vi "checkData.vi"(8 "error in (no error)":errorcluster, 11 "reference in":refnum<class "Notification Controller.lvclass">) -> (0 "error out":errorcluster, 3 "reference out":refnum<class "Notification Controller.lvclass">)   [LabVIEW 2014, in "Notification Controller.lvclass"]
uses:
  Notification Controller.lvclass
  APP/excelFile_class/fileType.ctl
  File Controller_llb/File Controller.lvclass
  APP/excelFile_class/excelFile.lvclass
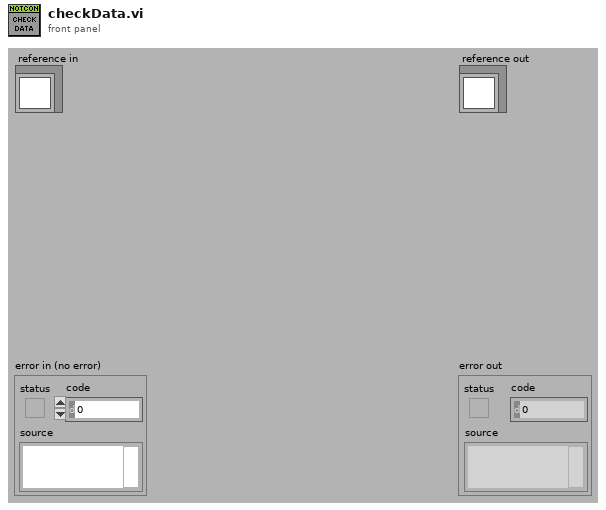
[diagram p1: front panel]
types:
  T1 = typedef "excelFile.lvclass/fileType.ctl" = enum16{"devices", "items", "partsTracking"}
  T2 = cluster{"second":i32, "minute":i32, "hour":i32, "day of month":i32, "month":i32, "year":i32, "day of week":i32, "day of year":i32, "is DST":i32}
  T3 = typedef "Notification Controller.lvclass/ObjectAttributesRef.ctl" = refnum<data-value>
  T4 = typedef "Notification Controller.lvclass/ObjectAttributes.ctl" = cluster{"MyAttribute":dbl, "items_data":string[][][], "items_notification_refs":refnum<class "itemsNotification.lvclass">[], "notifications_data_items":string[][], "items_nots?":bool, "devices_controller_ref":refnum<class "Devices Controller.lvclass">, "onlineUpdate":timestamp, "notController?":bool, "tracking_notification_ref":refnum<class "trackingNotification.lvclass">, "notifications_data_tracking":string[][], "tracking_parts_data":string[][], "tracking_nots?":bool, "index_tracking_not":i32[], "file_controller_ref":refnum<class "File Controller.lvclass">}
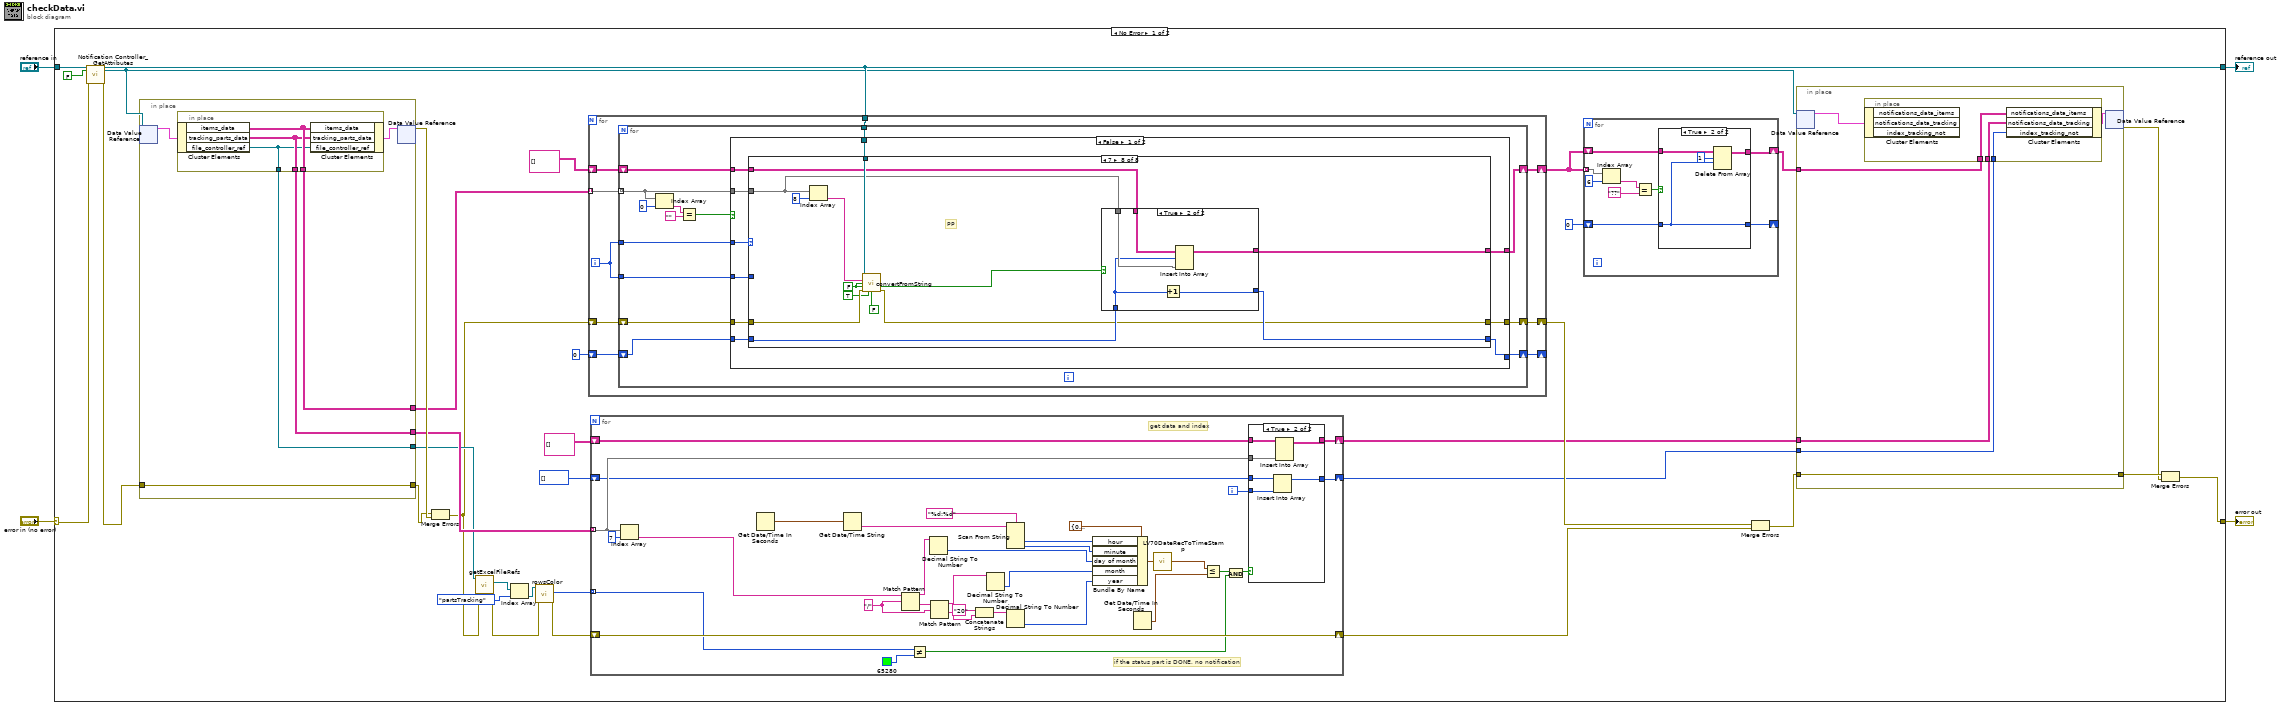
[diagram p0: block diagram]
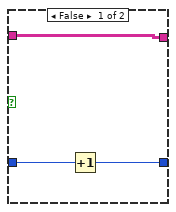
[diagram p3: hidden frame]
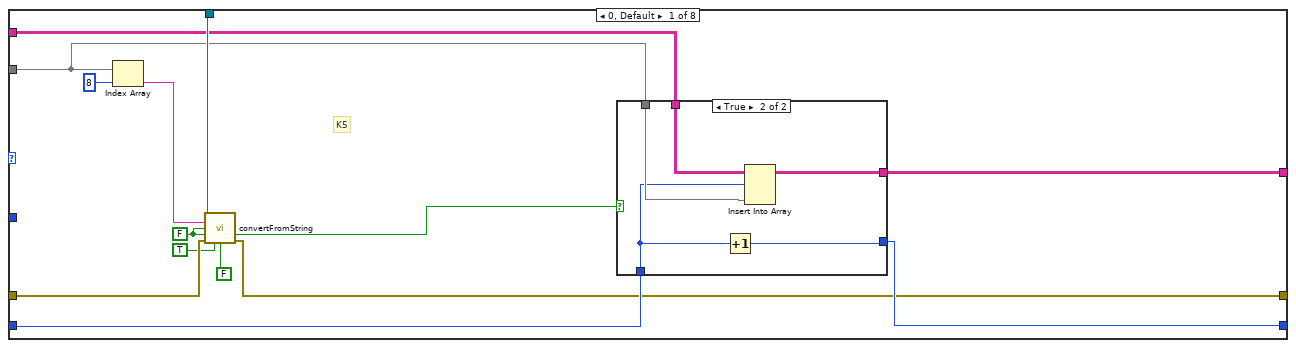
[diagram p4: hidden frame]
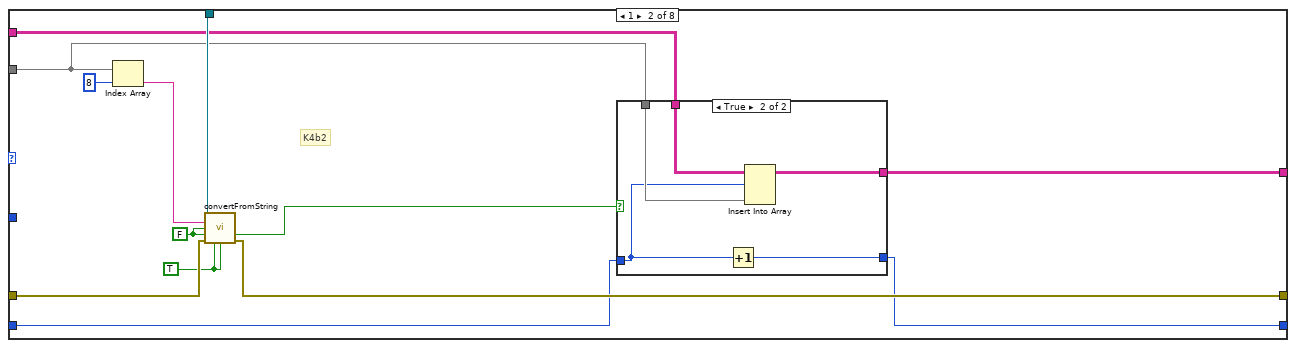
[diagram p6: hidden frame]
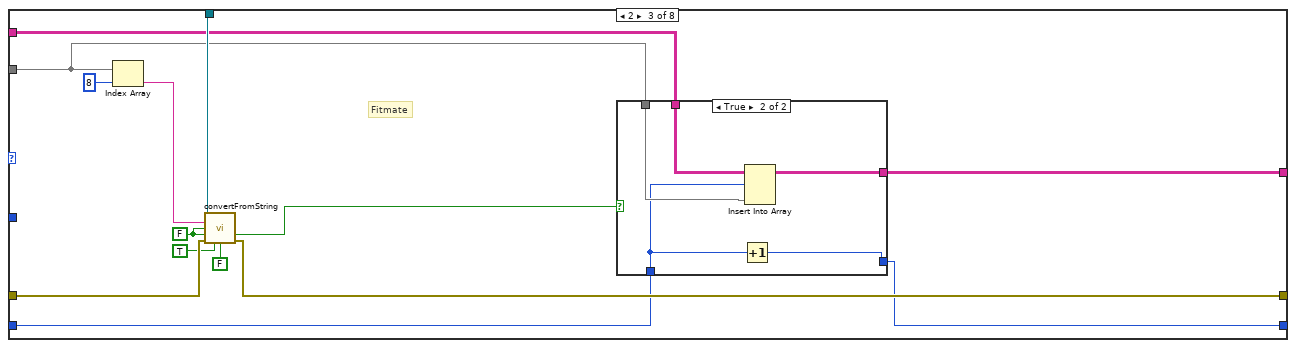
[diagram p8: hidden frame]
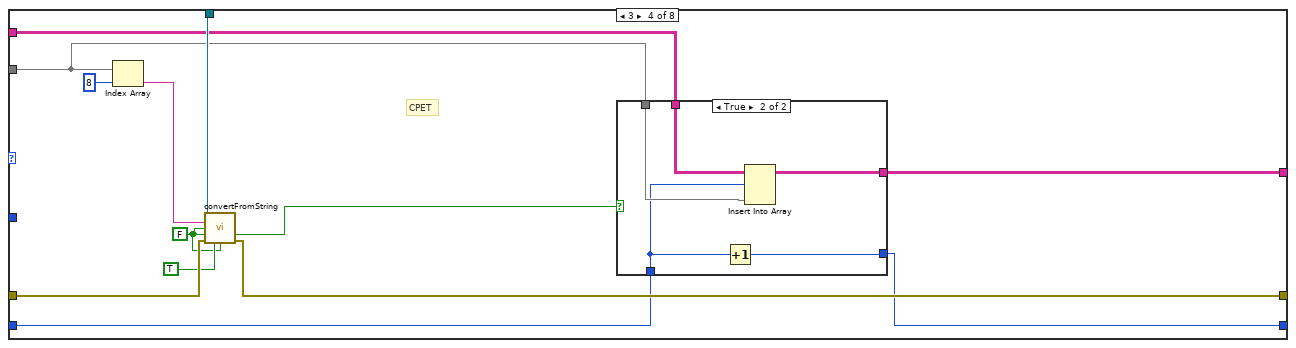
[diagram p10: hidden frame]
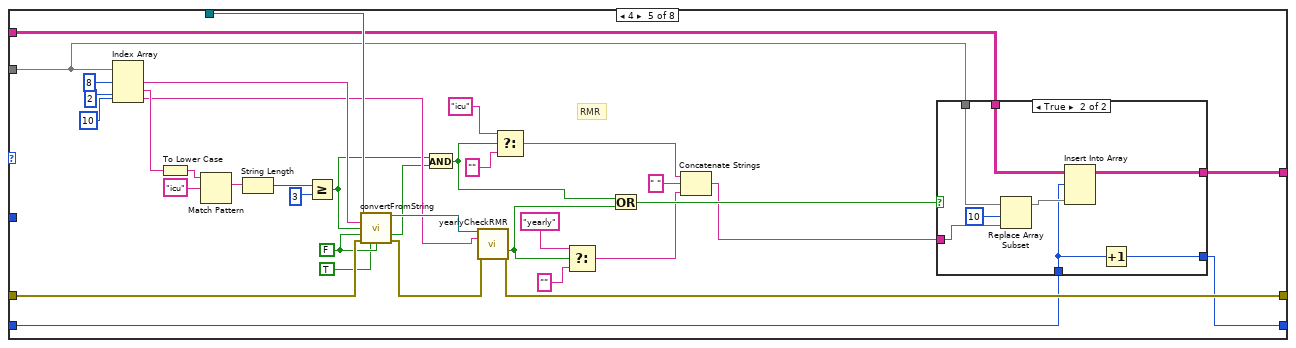
[diagram p12: hidden frame]
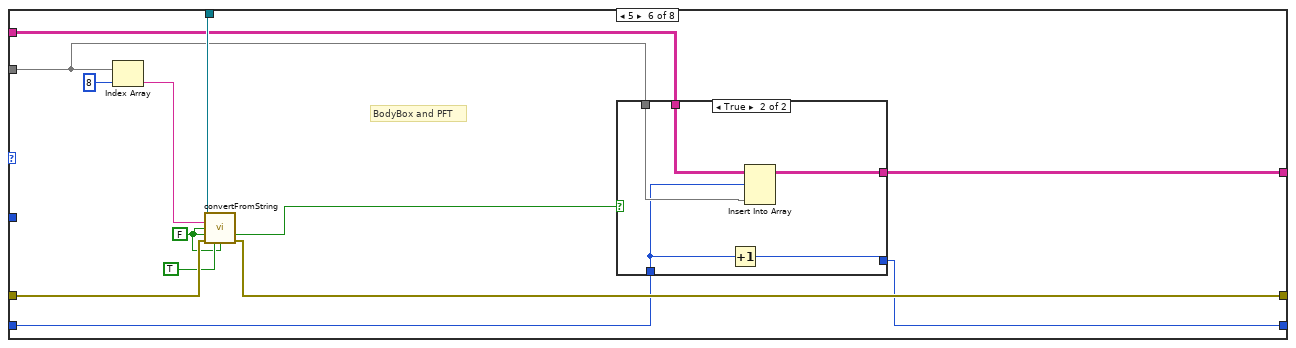
[diagram p14: hidden frame]
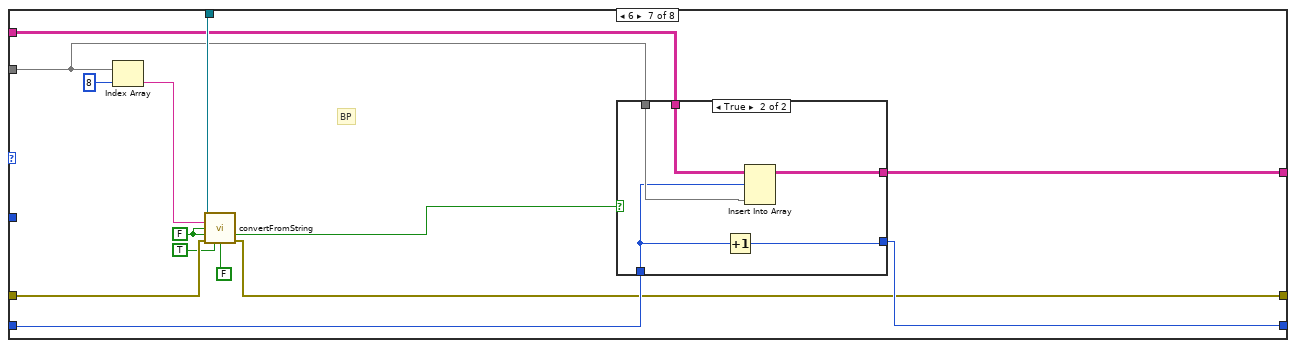
[diagram p16: hidden frame]
diagram:
  n1 = case shown="No Error" "error in (no error)" {
    selector: "error in (no error)" -> [w33 w340]
    tunnel: [w25 w340] -> w3
    tunnel: [w29 w339] -> w1
    tunnel: "reference in" -> [w35 w339]
    frame No Error {
      n2 = call "Notification Controller_GetAttributes.vi"("reference in"=w35, "return data? (T)"=FALSE, "error in (no error)"=w33) -> ("reference out"=w29:refnum<class "Notification Controller.lvclass">, "attributes ref"=w28:T3, "error out"=w32:errorcluster)  [unwired: 13 in, 1 out]
      n3 = in-place {
        in-place-border: w32 -> [w333]
        in-place-border: [w333] -> w36
        in-place-border: [w332] -> w30
        in-place-border: [w331] -> w20
        in-place-border: [w330] -> w12
        n4 = in-place-dvr #1(w28) -> (w334:T4)  [unwired: 1 out]
        n5 = in-place {
          in-place-border: [w338] -> w332
          in-place-border: [w337] -> w331
          in-place-border: [w336] -> w330
          n6 = in-place-cluster #2(w334) -> ("items_data"=w338:string[][][], "tracking_parts_data"=w337:string[][], "file_controller_ref"=w336:refnum<class "File Controller.lvclass">)
          n7 = in-place-cluster #2("items_data"=w338, "tracking_parts_data"=w337, "file_controller_ref"=w336) -> (w335:T4)
        }
        n8 = in-place-dvr #1(w335) -> (w37:errorcluster)  [unwired: 1 out]
      }
      n9 = Merge Errors(w36, w37) -> (w9:errorcluster)
      n10 = call "getExcelFileRefs.vi"("error in (no error)"=w9, "reference in"=w12) -> ("error out"=w5:errorcluster, "excelFile_refs"=w11:refnum<class "excelFile.lvclass">[])  [unwired: 7 in, 1 out]
      n11 = Index Array(array=w11, index=fileType."partsTracking" ("fileType")) -> (element=w8:refnum<class "excelFile.lvclass">)
      n12 = call "rowsColor.vi"("error in (no error)"=w5, "reference in"=w8) -> ("error out"=w7:errorcluster, "rowsColor"=w6:u32[])  [unwired: 7 in, 1 out]
      n13 = for {
        tunnel: w30 -> [w112] mode=indexing
        shift-right: [w109] -> w18
        shift-left: w9 -> [w111]
        tunnel: w29 -> [w108]
        shift-right: [w106] -> w23
        shift-left: string[][] [] ("data") -> [w107]
        shift-right: [w104] -> _
        shift-left: 0 -> [w105]
        i -> [w110]
        n14 = for {
          tunnel: w112 -> [w117] mode=indexing
          tunnel: w110 -> [w122]
          tunnel: w110 -> [w125]
          shift-right: [w123] -> w109
          shift-left: w111 -> [w126]
          tunnel: w108 -> [w124]
          shift-right: [w120] -> w106
          shift-left: w107 -> [w121]
          shift-right: [w118] -> w104
          shift-left: w105 -> [w119]
          n15 = Index Array(array=w117, index=0) -> (element=w114:string)
          n16 = Equal?(x=w114, y="") -> (x = y?=w113:bool)
          n17 = case shown="False" w113 {
            tunnel: w126 -> [w136 w328]
            tunnel: w125 -> [w135 _]
            tunnel: w124 -> [w134 _]
            tunnel: [w133 w328] -> w123
            tunnel: w122 -> [w132 _]
            tunnel: w121 -> [w131 w329]
            tunnel: [w130 w329] -> w120
            tunnel: w119 -> [w129 w327]
            tunnel: [w128 w327] -> w118
            tunnel: w117 -> [w127 _]
            frame False {
              n18 = case shown="7" w132 {
                tunnel: w136 -> [w150 w170 w191 w211 w254 w277 w298 w319]
                tunnel: w135 -> [_ _ _ _ _ _ _ _]
                tunnel: w127 -> [w144 w165 w185 w206 w249 w272 w292 w313]
                tunnel: w134 -> [w148 w168 w189 w209 w252 w275 w296 w317]
                tunnel: [w138 w163 w183 w204 w239 w270 w286 w307] -> w133
                tunnel: w131 -> [w145 w166 w186 w207 w250 w273 w293 w314]
                tunnel: [w143 w164 w184 w205 w248 w271 w291 w312] -> w130
                tunnel: w129 -> [w141 w161 w181 w201 w228 w267 w289 w310]
                tunnel: [w140 w160 w180 w200 w227 w266 w288 w309] -> w128
                frame 0, Default {
                  w146 = FALSE ("getDate")
                  # "K5"
                  n19 = Index Array(array=w144, index=8) -> (element=w149:string)
                  n20 = call "convertFromString.vi"("reference in"=w148, "dateString"=w149, "ICU?"=w146, "getDate"=w146, "error in (no error)"=w150, "yearly?"=TRUE ("k4b2?"), "k4b2?"=FALSE) -> ("send?"=w137:bool, "error out"=w138:errorcluster)  [unwired: 5 in, 2 out]
                  n21 = case shown="True" w137 {
                    tunnel: w145 -> [w152 w157]
                    tunnel: w144 -> [_ w156]
                    tunnel: [w152 w155] -> w143
                    tunnel: w141 -> [w151 w154]
                    tunnel: [w151 w153] -> w140
                    frame False {
                    }
                    frame True {
                      n22 = Increment(x=w154) -> (x+1=w153:i32)
                      n23 = Insert Into Array(array=w157, index (row)=w154, new element=w156) -> (w155:string[][])  [unwired: 1 in]
                    }
                  }
                }
                frame 1 {
                  w158 = TRUE ("k4b2?")
                  w159 = FALSE ("getDate")
                  # "K4b2"
                  n24 = Index Array(array=w165, index=8) -> (element=w169:string)
                  n25 = call "convertFromString.vi"("reference in"=w168, "dateString"=w169, "ICU?"=w159, "getDate"=w159, "error in (no error)"=w170, "yearly?"=w158, "k4b2?"=w158) -> ("send?"=w162:bool, "error out"=w163:errorcluster)  [unwired: 5 in, 2 out]
                  n26 = case shown="True" w162 {
                    tunnel: w166 -> [w172 w177]
                    tunnel: w165 -> [_ w176]
                    tunnel: [w172 w175] -> w164
                    tunnel: w161 -> [w171 w174]
                    tunnel: [w171 w173] -> w160
                    frame False {
                    }
                    frame True {
                      n27 = Increment(x=w174) -> (x+1=w173:i32)
                      n28 = Insert Into Array(array=w177, index (row)=w174, new element=w176) -> (w175:string[][])  [unwired: 1 in]
                    }
                  }
                }
                frame 2 {
                  w187 = FALSE ("getDate")
                  # "Fitmate"
                  n29 = Index Array(array=w185, index=8) -> (element=w190:string)
                  n30 = call "convertFromString.vi"("reference in"=w189, "dateString"=w190, "ICU?"=w187, "getDate"=w187, "error in (no error)"=w191, "yearly?"=TRUE, "k4b2?"=FALSE) -> ("send?"=w182:bool, "error out"=w183:errorcluster)  [unwired: 5 in, 2 out]
                  n31 = case shown="True" w182 {
                    tunnel: w186 -> [w193 w198]
                    tunnel: w185 -> [_ w197]
                    tunnel: [w193 w196] -> w184
                    tunnel: w181 -> [w192 w195]
                    tunnel: [w192 w194] -> w180
                    frame False {
                    }
                    frame True {
                      n32 = Increment(x=w195) -> (x+1=w194:i32)
                      n33 = Insert Into Array(array=w198, index (row)=w195, new element=w197) -> (w196:string[][])  [unwired: 1 in]
                    }
                  }
                }
                frame 3 {
                  w199 = FALSE ("getDate")
                  # "CPET"
                  n34 = Index Array(array=w206, index=8) -> (element=w210:string)
                  n35 = call "convertFromString.vi"("reference in"=w209, "dateString"=w210, "ICU?"=w199, "getDate"=w199, "error in (no error)"=w211, "yearly?"=TRUE ("k4b2?"), "k4b2?"=w199) -> ("send?"=w203:bool, "error out"=w204:errorcluster)  [unwired: 5 in, 2 out]
                  n36 = case shown="True" w203 {
                    tunnel: w207 -> [w213 w218]
                    tunnel: w206 -> [_ w217]
                    tunnel: [w213 w216] -> w205
                    tunnel: w201 -> [w212 w215]
                    tunnel: [w212 w214] -> w200
                    frame False {
                    }
                    frame True {
                      n37 = Increment(x=w215) -> (x+1=w214:i32)
                      n38 = Insert Into Array(array=w218, index (row)=w215, new element=w217) -> (w216:string[][])  [unwired: 1 in]
                    }
                  }
                }
                frame 4 {
                  w224 = FALSE ("k4b2?")
                  # "RMR"
                  n39 = Index Array(array=w249, index #1=8 ("index"), index #2=2 ("index"), index #3=10 ("index")) -> (element #1=w253:string, element #2=w241:string, element #3=w225:string)
                  n40 = To Lower Case(string=w241) -> (all lower case string=w247:string)
                  n41 = Match Pattern(string=w247, regular expression="icu") -> (match substring=w245:string)  [unwired: 1 in, 3 out]
                  n42 = String Length(string=w245) -> (length=w244:i32)
                  n43 = Greater Or Equal?(x=w244, y=3) -> (x >= y?=w222:bool)
                  n44 = call "convertFromString.vi"("reference in"=w252, "dateString"=w253, "ICU?"=w222, "getDate"=w224, "error in (no error)"=w254, "yearly?"=TRUE, "k4b2?"=w224) -> ("reference out"=w238:refnum<class "Notification Controller.lvclass">, "send?"=w221:bool, "error out"=w240:errorcluster)  [unwired: 5 in, 1 out]
                  n45 = And(x=w222, y=w221) -> (x .and. y?=w220:bool)
                  n46 = call "yearlyCheckRMR.vi"("reference in"=w238, "dateString"=w225, "error in (no error)"=w240) -> ("send?"=w219:bool, "error out"=w239:errorcluster)  [unwired: 10 in, 1 out]
                  n47 = Select(t="icu", s=w220, f="") -> (s? t:f=w230:string)
                  n48 = Select(t="yearly", s=w219, f="") -> (s? t:f=w232:string)
                  n49 = Or(x=w220, y=w219) -> (x .or. y?=w235:bool)
                  n50 = Concatenate Strings(w230, " " ("string"), w232) -> (w229:string)
                  n51 = case shown="True" w235 {
                    tunnel: w250 -> [w256 w264]
                    tunnel: w249 -> [_ w262]
                    tunnel: [w256 w263] -> w248
                    tunnel: w229 -> [_ w261]
                    tunnel: w228 -> [w255 w258]
                    tunnel: [w255 w257] -> w227
                    frame False {
                    }
                    frame True {
                      n52 = Replace Array Subset(array=w262, new element=w261, index=10) -> (w260:string[])
                      n53 = Insert Into Array(array=w264, index (row)=w258, new element=w260) -> (w263:string[][])  [unwired: 1 in]
                      n54 = Increment(x=w258) -> (x+1=w257:i32)
                    }
                  }
                }
                frame 5 {
                  w265 = FALSE ("getDate")
                  # "BodyBox and PFT"
                  n55 = Index Array(array=w272, index=8) -> (element=w276:string)
                  n56 = call "convertFromString.vi"("reference in"=w275, "dateString"=w276, "ICU?"=w265, "getDate"=w265, "error in (no error)"=w277, "yearly?"=TRUE ("k4b2?"), "k4b2?"=w265) -> ("send?"=w269:bool, "error out"=w270:errorcluster)  [unwired: 5 in, 2 out]
                  n57 = case shown="True" w269 {
                    tunnel: w273 -> [w279 w284]
                    tunnel: w272 -> [_ w283]
                    tunnel: [w279 w282] -> w271
                    tunnel: w267 -> [w278 w281]
                    tunnel: [w278 w280] -> w266
                    frame False {
                    }
                    frame True {
                      n58 = Increment(x=w281) -> (x+1=w280:i32)
                      n59 = Insert Into Array(array=w284, index (row)=w281, new element=w283) -> (w282:string[][])  [unwired: 1 in]
                    }
                  }
                }
                frame 6 {
                  w294 = FALSE ("getDate")
                  # "BP"
                  n60 = Index Array(array=w292, index=8) -> (element=w297:string)
                  n61 = call "convertFromString.vi"("reference in"=w296, "dateString"=w297, "ICU?"=w294, "getDate"=w294, "error in (no error)"=w298, "yearly?"=TRUE ("k4b2?"), "k4b2?"=FALSE) -> ("send?"=w285:bool, "error out"=w286:errorcluster)  [unwired: 5 in, 2 out]
                  n62 = case shown="True" w285 {
                    tunnel: w293 -> [w300 w305]
                    tunnel: w292 -> [_ w304]
                    tunnel: [w300 w303] -> w291
                    tunnel: w289 -> [w299 w302]
                    tunnel: [w299 w301] -> w288
                    frame False {
                    }
                    frame True {
                      n63 = Increment(x=w302) -> (x+1=w301:i32)
                      n64 = Insert Into Array(array=w305, index (row)=w302, new element=w304) -> (w303:string[][])  [unwired: 1 in]
                    }
                  }
                }
                frame 7 {
                  w315 = FALSE ("getDate")
                  # "PP"
                  n65 = Index Array(array=w313, index=8) -> (element=w318:string)
                  n66 = call "convertFromString.vi"("reference in"=w317, "dateString"=w318, "ICU?"=w315, "getDate"=w315, "error in (no error)"=w319, "yearly?"=TRUE ("k4b2?"), "k4b2?"=FALSE) -> ("send?"=w306:bool, "error out"=w307:errorcluster)  [unwired: 5 in, 2 out]
                  n67 = case shown="True" w306 {
                    tunnel: w314 -> [w321 w326]
                    tunnel: w313 -> [_ w325]
                    tunnel: [w321 w324] -> w312
                    tunnel: w310 -> [w320 w323]
                    tunnel: [w320 w322] -> w309
                    frame False {
                    }
                    frame True {
                      n68 = Increment(x=w323) -> (x+1=w322:i32)
                      n69 = Insert Into Array(array=w326, index (row)=w323, new element=w325) -> (w324:string[][])  [unwired: 1 in]
                    }
                  }
                }
              }
            }
            frame True {
            }
          }
        }
      }
      n70 = for {
        tunnel: w20 -> [w46] mode=indexing
        shift-right: [w50] -> w16
        shift-left: w7 -> [w50]
        shift-right: [w47] -> w15
        shift-left: string[][] [] ("data") -> [w48]
        shift-right: [w43] -> w13
        shift-left: i32[] [] -> [w44]
        tunnel: w6 -> [w40] mode=indexing
        i -> [w42]
        w63 = "/" ("regular expression")
        # "if the status part is DONE, no notification"
        # "get data and index"
        n71 = Index Array(array=w46, index=7) -> (element=w53:string)
        n72 = Get Date/Time In Seconds() -> (seconds since 1Jan1904=w70:timestamp)
        n73 = Get Date/Time String(seconds (now)=w70) -> (time string=w64:string)  [unwired: 3 out]
        n74 = Match Pattern(string=w53, regular expression=w63) -> (before substring=w61:string, after substring=w60:string)  [unwired: 1 in, 2 out]
        n75 = Not Equal?(x=w40, y=u32 65280) -> (x != y?=w38:bool)
        n76 = Decimal String To Number(string=w61) -> (number=w62:i32)  [unwired: 2 in, 1 out]
        n77 = Match Pattern(string=w60, regular expression=w63) -> (before substring=w52:string, after substring=w55:string)  [unwired: 1 in, 2 out]
        n78 = Concatenate Strings("20" ("string"), w55) -> (w57:string)
        n79 = Decimal String To Number(string=w52) -> (number=w51:i32)  [unwired: 2 in, 1 out]
        n80 = Scan From String "Scan From String"(format string="%d:%d", input string=w64) -> (output 1=w66:i32, output 2=w65:i32)  [unwired: 4 in, 3 out]
        n81 = Decimal String To Number(string=w57) -> (number=w45:i32)  [unwired: 2 in, 1 out]
        n82 = Bundle By Name(cluster=T2 {"second"=0, "minute"=0, "hour"=0, "day of month"=0, "month"=0, "year"=0, "day of week"=0, "day of year"=0, "is DST"=0} ("date time rec"), "hour"=w66, "minute"=w65, "day of month"=w62, "month"=w51, "year"=w45) -> (w67:T2)
        n83 = Get Date/Time In Seconds() -> (seconds since 1Jan1904=w58:timestamp)
        n84 = call <vilib>:"LV70DateRecToTimeStamp.vi"("date time rec"=w67) -> ("Time Stamp"=w59:timestamp)
        n85 = Less Or Equal?(x=w59, y=w58) -> (x <= y?=w49:bool)
        n86 = And(x=w49, y=w38) -> (x .and. y?=w41:bool)
        n87 = case shown="True" w41 {
          tunnel: w48 -> [w72 w78]
          tunnel: [w72 w76] -> w47
          tunnel: w46 -> [_ w77]
          tunnel: w44 -> [w71 w75]
          tunnel: [w71 w74] -> w43
          tunnel: w42 -> [_ w73]
          frame False {
          }
          frame True {
            n88 = Insert Into Array(array=w75, new element=w73) -> (w74:i32[])  [unwired: 1 in]
            n89 = Insert Into Array(array=w78, new element=w77) -> (w76:string[][])  [unwired: 2 in]
          }
        }
      }
      n90 = for {
        tunnel: w23 -> [w87] mode=indexing
        shift-right: [w82] -> w22
        shift-left: w23 -> [w83]
        shift-right: [w79] -> _
        shift-left: 0 ("index") -> [w80]
        n91 = Index Array(array=w87, index=6) -> (element=w85:string)
        n92 = Equal?(x=w85, y="??") -> (x = y?=w81:bool)
        n93 = case shown="True" w81 {
          tunnel: w83 -> [w89 w94]
          tunnel: [w89 w93] -> w82
          tunnel: [w88 w91] -> w79
          tunnel: w80 -> [w90 w91]
          frame False {
            n94 = Increment(x=w90) -> (x+1=w88:i32)
          }
          frame True {
            n95 = Delete From Array(array=w94, length=1, index (row)=w91) -> (array with subset deleted=w93:string[][])  [unwired: 1 in, 1 out]
          }
        }
      }
      n96 = Merge Errors(w18, w16) -> (w17:errorcluster)
      n97 = in-place {
        in-place-border: w17 -> [w98]
        in-place-border: [w98] -> w27
        in-place-border: w22 -> [w97]
        in-place-border: w15 -> [w96]
        in-place-border: w13 -> [w95]
        n98 = in-place-dvr #3(w28) -> (w99:T4)  [unwired: 1 out]
        n99 = in-place {
          in-place-border: w97 -> [w103]
          in-place-border: w96 -> [w102]
          in-place-border: w95 -> [w101]
          n100 = in-place-cluster #4(w99) -> ()  [unwired: 3 out]
          n101 = in-place-cluster #4("notifications_data_items"=w103, "notifications_data_tracking"=w102, "index_tracking_not"=w101) -> (w100:T4)
        }
        n102 = in-place-dvr #3(w100) -> (w26:errorcluster)  [unwired: 1 out]
      }
      n103 = Merge Errors(w27, w26) -> (w25:errorcluster)
    }
    frame Error {
    }
  }
  "error out" <- w3
  "reference out" <- w1
